vi "MC5e Squad_Editor.vi"(6 "Mode":T1, 8 "error in":errorcluster, 11 "index":i32) -> (0 "error out":errorcluster, 2 "Cancelled":bool)   [LabVIEW 2020]
uses:
  MC5e Squad_Info.ctl
  MC5e Size_Categories.ctl
  MC53 Sqad_editor_modes.ctl
  MC5e Squad_Manager_Modes.ctl
panel:
  in  "OK Button":bool
  in  "Cancel Button":bool
  in  "Squad In":T2={"Squad Name"="", "# Soldiers"=1, "Battle Rating"=0, "Flying"=FALSE, "Mounted"=FALSE, "Speed"=3, "Range"=1, "Morale"=0, "Token Image"=variant, "Max Endurance"=10, "Current Endurance"=10, "Size"=enum."Medium", "Space Taken"=1, "Difficult Terrain"=[0, 1, 3, 6, 7], "CR"=1, "Special / Notes"=""} {"CR" items=["1/8", "1/4", "1/2", "1", "2", "3", "4", "5", "6", "7", "8", "9", "10", "11", "12", "13", "14", "15", "16", "17", "18", "19", "20", "21", "22", "23", "24", "25", "26", "27", "28", "29", "30"]}
  # "Squads are restricted to one type of soldier (i.e  Archers) and all of the same level.\nIf you want mixed CR or mixed types, use multiple squads."
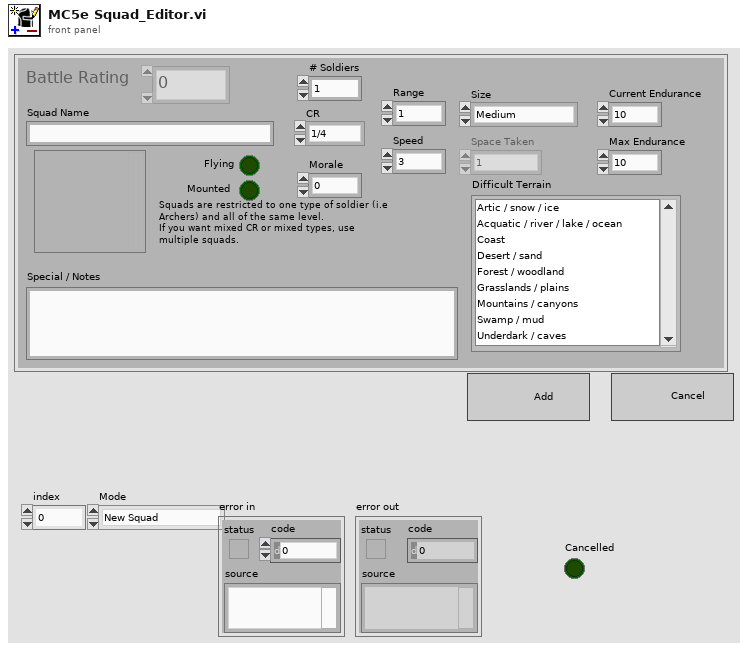
[diagram p1: front panel]
types:
  T1 = typedef "MC53 Sqad_editor_modes.ctl" = enum16{"New Squad", "Copy Squad", "Delete Squad", "Edit Squad"}
  T2 = typedef "MC5e Squad_Info.ctl" = cluster{"Squad Name":string, "# Soldiers":u16, "Battle Rating":u16, "Flying":bool, "Mounted":bool, "Speed":u16, "Range":u16, "Morale":i32, "Token Image":variant, "Max Endurance":u16, "Current Endurance":i32, "Size":T3, "Space Taken":u16, "Difficult Terrain":i32[], "CR":u16, "Special / Notes":string}
  T3 = typedef "MC5e Size_Categories.ctl" = enum16{"Tiny", "Small", "Medium", "Large", "Huge", "Gargantuan"}
  T4 = enum8{"Enabled", "Disabled", "Disabled and Grayed Out"}
  T5 = typedef "MC5e Squad_Manager_Modes.ctl" = enum16{"Initialize", "Add Squad", "Delete Squad", "Get Squad"}
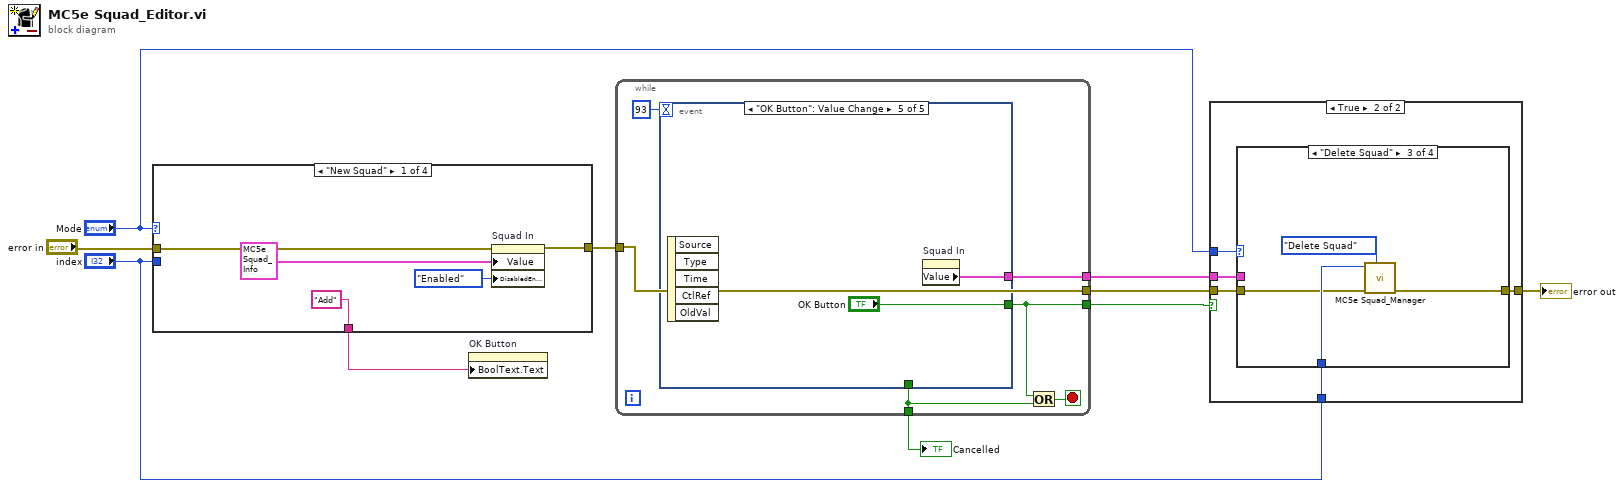
[diagram p0: block diagram]
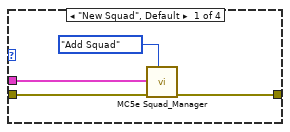
[diagram p3: hidden frame]
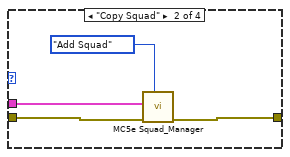
[diagram p4: hidden frame]
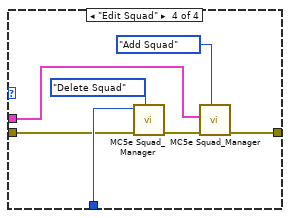
[diagram p5: hidden frame]
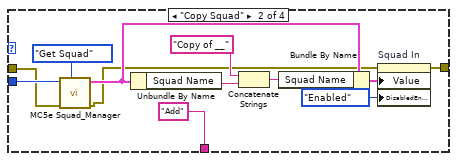
[diagram p6: hidden frame]
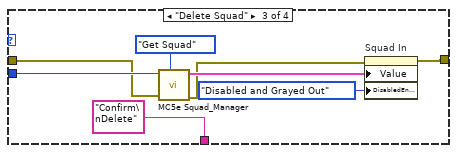
[diagram p7: hidden frame]
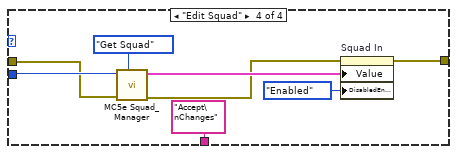
[diagram p8: hidden frame]
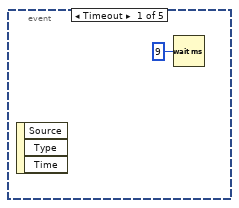
[diagram p9: hidden frame]
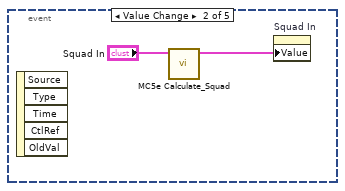
[diagram p10: hidden frame]
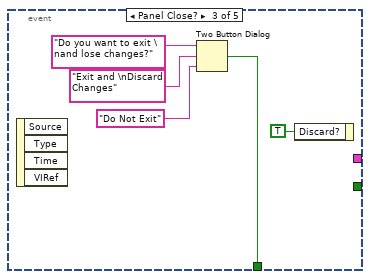
[diagram p11: hidden frame]
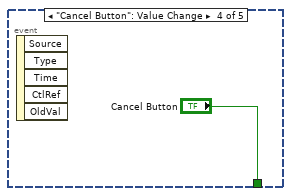
[diagram p12: hidden frame]
diagram:
  n1 = case shown="\"New Squad\"" "Mode" {
    tunnel: "index" -> [_ w27 w33 w42]
    tunnel: ["Add" ("Caption.Text") "Add" ("Caption.Text") "Confirm\nDelete" ("Caption.Text") "Accept\nChanges" ("Caption.Text")] -> w10
    tunnel: [w13 w19 w31 w39] -> w9
    tunnel: "error in" -> [w11 w17 w29 w37]
    frame "New Squad" {
      n2 = property on="Squad In" class="Clust (strict)"(error in=w11, "Value"=T2 {"Squad Name"="", "# Soldiers"=1, "Battle Rating"=0, "Flying"=FALSE, "Mounted"=FALSE, "Speed"=3, "Range"=1, "Morale"=0, "Token Image"=variant, "Max Endurance"=10, "Current Endurance"=10, "Size"=enum."Medium", "Space Taken"=1, "Difficult Terrain"=[0, 1, 3, 6, 7], "CR"=1, "Special / Notes"=""} ("Squad In"), "DisabledEnum"=T4."Enabled" ("Disabled")) -> (error out=w13:errorcluster)  [unwired: 1 in, 1 out]
    }
    frame "Copy Squad" {
      n3 = call "MC5e Squad_Manager.vi"("Mode"=MC5e_Squad_Manager_Modes."Get Squad", "error in"=w17, "index (get/delete)"=w27) -> ("error out"=w16:errorcluster, "Squad"=w22:T2)  [unwired: 5 in, 2 out]
      n4 = Unbundle By Name(w22) -> ("Squad Name"=w25:string)
      n5 = Concatenate Strings("Copy of __" ("string"), w25) -> (w23:string)
      n6 = Bundle By Name(cluster=w22, "Squad Name"=w23) -> (w21:T2)
      n7 = property on="Squad In" class="Clust (strict)"(error in=w16, "Value"=w21, "DisabledEnum"=T4."Enabled" ("Disabled")) -> (error out=w19:errorcluster)  [unwired: 1 in, 1 out]
    }
    frame "Delete Squad" {
      n8 = call "MC5e Squad_Manager.vi"("Mode"=MC5e_Squad_Manager_Modes."Get Squad", "error in"=w29, "index (get/delete)"=w33) -> ("error out"=w28:errorcluster, "Squad"=w35:T2)  [unwired: 5 in, 2 out]
      n9 = property on="Squad In" class="Clust (strict)"(error in=w28, "Value"=w35, "DisabledEnum"=T4."Disabled and Grayed Out" ("Disabled")) -> (error out=w31:errorcluster)  [unwired: 1 in, 1 out]
    }
    frame "Edit Squad" {
      n10 = call "MC5e Squad_Manager.vi"("Mode"=MC5e_Squad_Manager_Modes."Get Squad", "error in"=w37, "index (get/delete)"=w42) -> ("error out"=w36:errorcluster, "Squad"=w41:T2)  [unwired: 5 in, 2 out]
      n11 = property on="Squad In" class="Clust (strict)"(error in=w36, "Value"=w41, "DisabledEnum"=T4."Enabled" ("Disabled")) -> (error out=w39:errorcluster)  [unwired: 1 in, 1 out]
    }
  }
  n12 = property on="OK Button" class="Bool"("BoolText.Text"=w10) -> ()  [unwired: 2 in, 2 out]
  n13 = while {
    tunnel: [w45] -> w7
    tunnel: w9 -> [w48]
    tunnel: [w48] -> w3
    tunnel: [w47] -> w2
    tunnel: [w44] -> w1
    stop <- w46 stop-if-true
    n14 = event shown="[4] \"OK Button\": Value Change" {
      selector: _ -> [_ _ _ _ _]
      dyn-events: _ -> [_ _ _ _ _]
      timeout: 93 -> [_ _ _ _ _]
      tunnel: [_ _ w53 "Cancel Button" _] -> w47
      tunnel: [_ _ _ _ "OK Button"] -> w45
      tunnel: [_ _ _ _ w59] -> w44
      event Timeout {
        n15 = event-data() -> ()  [unwired: 1 in, 3 out]
        n16 = Wait (ms)(milliseconds to wait=u32 9) -> ()  [unwired: 1 out]
      }
      event Value Change {
        n17 = event-data() -> ()  [unwired: 1 in, 5 out]
        n18 = call "MC5e Calculate_Squad.vi"("Input Squad"="Squad In") -> ("output squad"=w51:T2)  [unwired: 10 in]
        n19 = property on="Squad In" class="Clust (strict)"("Value"=w51) -> ()  [unwired: 2 in, 2 out]
      }
      event Panel Close? {
        n20 = event-data() -> ()  [unwired: 1 in, 4 out]
        n21 = Two Button Dialog(message="Do you want to exit \nand lose changes?", 1:"Do Not Exit" ("F button name (\"Cancel\")"), 2:"Exit and \nDiscard Changes" ("T button name (\"OK\")")) -> (T button?=w53:bool)
        n22 = event-data("Discard?"=TRUE) -> ()  [unwired: 1 in, 1 out]
      }
      event "Cancel Button": Value Change {
        n23 = event-data() -> ()  [unwired: 1 in, 5 out]
      }
      event "OK Button": Value Change {
        n24 = event-data() -> ()  [unwired: 1 in, 5 out]
        n25 = property on="Squad In" class="Clust (strict)"() -> ("Value"=w59:T2)  [unwired: 2 in, 2 out]
      }
    }
    n26 = Or(x=w45, y=w47) -> (x .or. y?=w46:bool)
  }
  "Cancelled" <- w2
  n27 = case shown="True" w7 {
    tunnel: "Mode" -> [_ w65]
    tunnel: "index" -> [_ w64]
    tunnel: [_ w63] -> w5
    tunnel: w3 -> [_ w62]
    tunnel: w1 -> [_ w61]
    frame False {
    }
    frame True {
      n28 = case shown="\"Delete Squad\"" w65 {
        tunnel: w64 -> [_ _ w76 w80]
        tunnel: [w68 w72 w75 w81] -> w63
        tunnel: w62 -> [w67 w71 w74 w78]
        tunnel: w61 -> [w66 w70 _ w79]
        frame "New Squad", Default {
          n29 = call "MC5e Squad_Manager.vi"("Mode"=MC5e_Squad_Manager_Modes."Add Squad", "error in"=w67, "Squad In (Add/Replace)"=w66) -> ("error out"=w68:errorcluster)  [unwired: 5 in, 3 out]
        }
        frame "Copy Squad" {
          n30 = call "MC5e Squad_Manager.vi"("Mode"=MC5e_Squad_Manager_Modes."Add Squad", "error in"=w71, "Squad In (Add/Replace)"=w70) -> ("error out"=w72:errorcluster)  [unwired: 5 in, 3 out]
        }
        frame "Delete Squad" {
          n31 = call "MC5e Squad_Manager.vi"("Mode"=MC5e_Squad_Manager_Modes."Delete Squad", "error in"=w74, "index (get/delete)"=w76) -> ("error out"=w75:errorcluster)  [unwired: 5 in, 3 out]
        }
        frame "Edit Squad" {
          n32 = call "MC5e Squad_Manager.vi"("Mode"=MC5e_Squad_Manager_Modes."Delete Squad", "error in"=w78, "index (get/delete)"=w80) -> ("error out"=w83:errorcluster)  [unwired: 5 in, 3 out]
          n33 = call "MC5e Squad_Manager.vi"("Mode"=MC5e_Squad_Manager_Modes."Add Squad", "error in"=w83, "Squad In (Add/Replace)"=w79) -> ("error out"=w81:errorcluster)  [unwired: 5 in, 3 out]
        }
      }
    }
  }
  "error out" <- w5
